vi "Check If Pixels Belong In Sector.vi"() -> (3 "FIFO Timeout?":bool)   [LabVIEW 2013]
uses:
  Globals/Pixel Location Global.vi
  Globals/Accumulated Sector Intensity.vi
  Globals/Sector Parameter Global.vi
  <vilib>/rvi/FIFO/Fifo_Resource/nirvififoEmulationReadFpgaImpl.vi
  <vilib>/rvi/DataTransferAndStorage/Container/Common/niFpgaContainerGetUniqueNameForEmu.vi
  <vilib>/rvi/FIFO/Fifo_Resource/nirvififoEmulationWriteFpgaImpl.vi
  <vilib>/rvi/DataTransferAndStorage/Container/XNode/niFpgaContainer.xnode
  <vilib>/rvi/FIFO/Fifo_Resource/nirvififoEmulationRead.vi
  <vilib>/rvi/FIFO/Fifo_Resource/nirvififoEmulationWrite.vi
panel:
  out "End of  Data?":bool
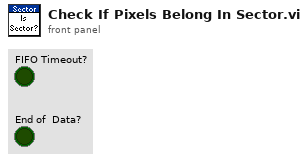
[diagram p1: front panel]
types:
  T1 = cluster{"Pixel Value":u8, "X":fxp<+,11,11>, "Y":fxp<+,11,11>}
  T2 = typedef "Sector Parameter Cluster.ctl" = cluster{"Start Angle":fxp<+/-,17,2>, "End Angle":fxp<+/-,17,2>, "Inner Radius":u16, "Outter Radius":u16, "Hinge X":u16, "Hinge Y":u16, "NumWingSectors":u8}
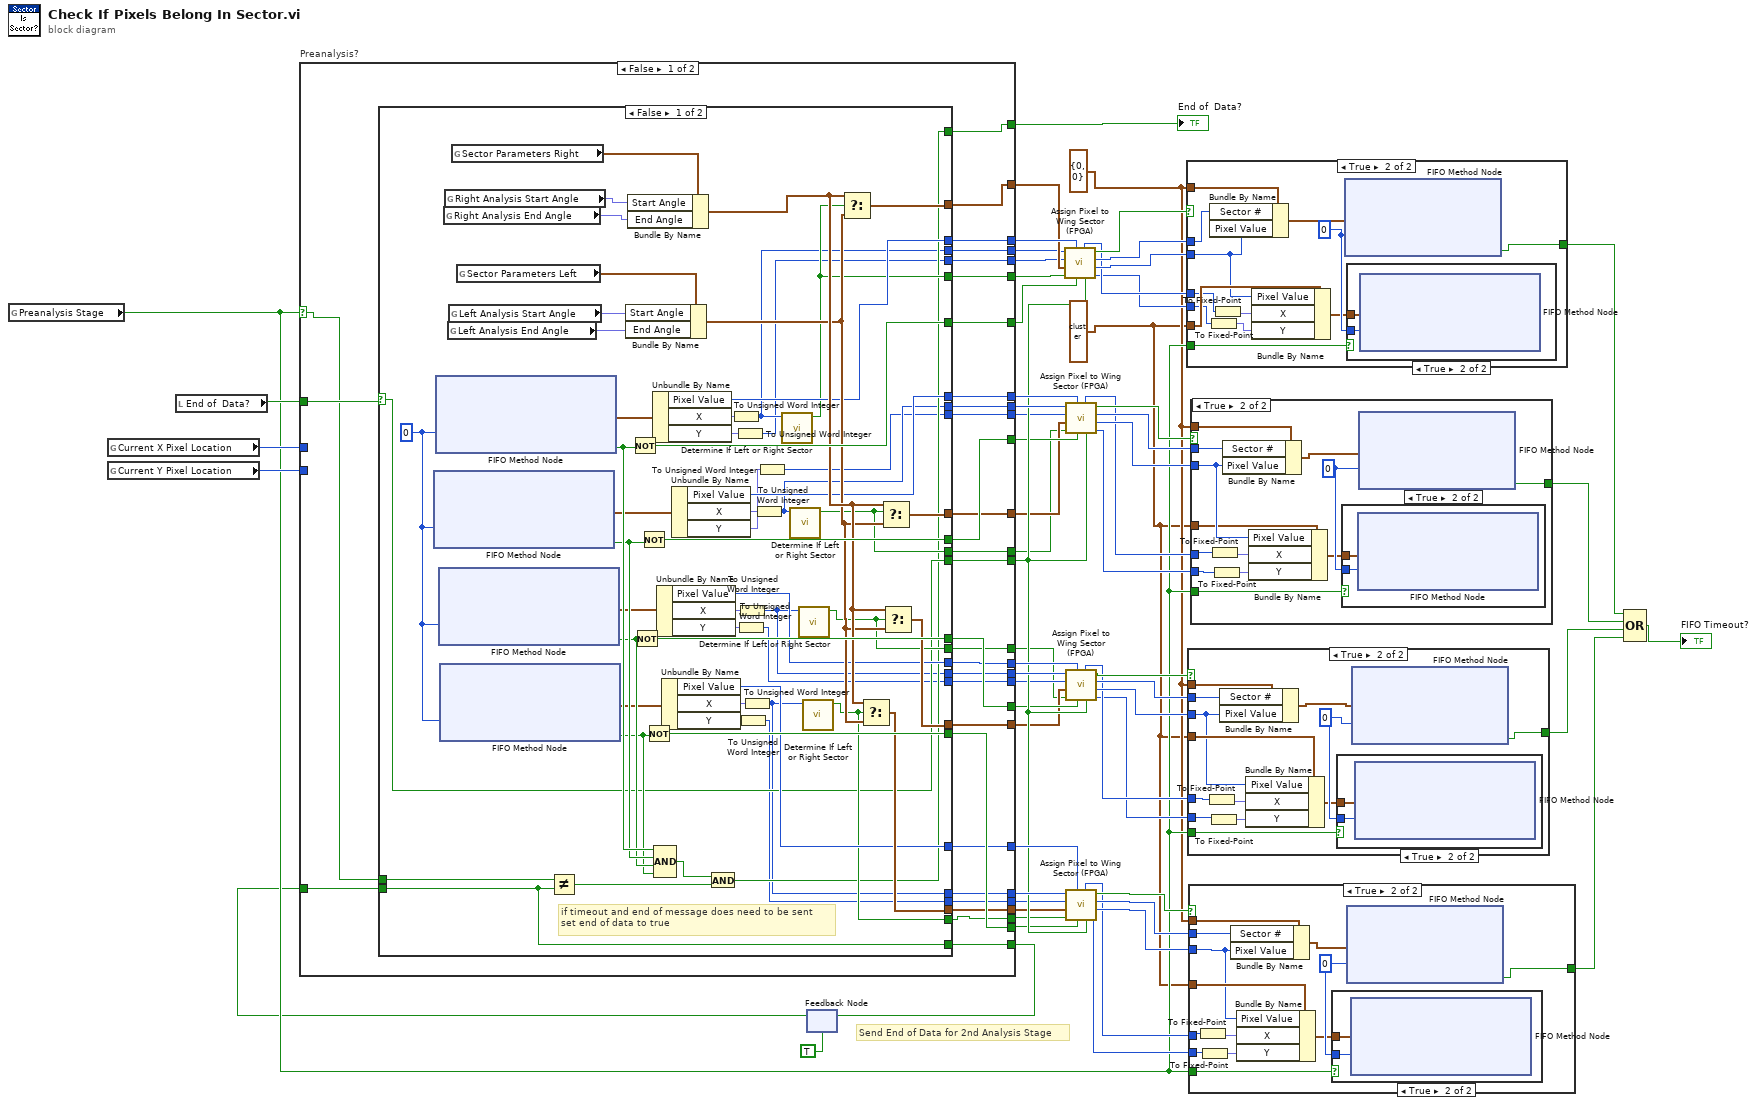
[diagram p0: block diagram]
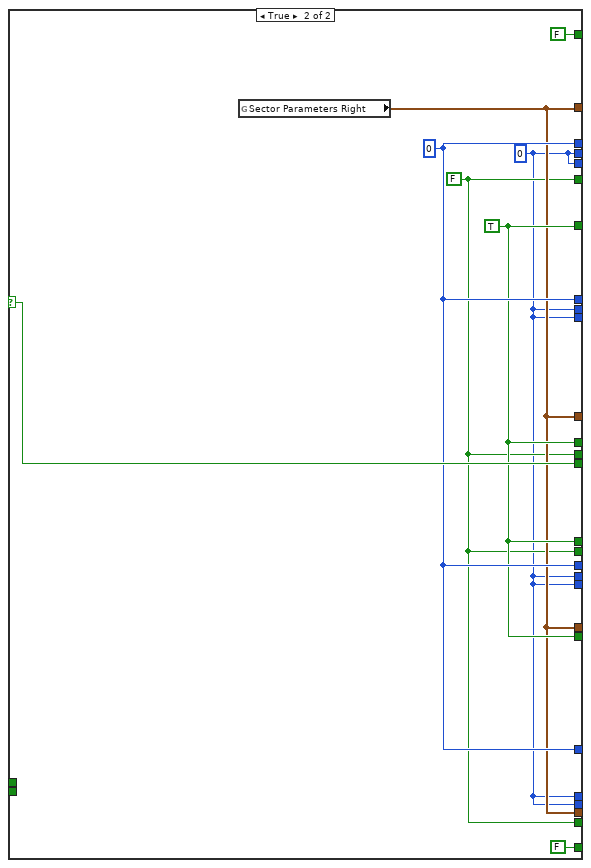
[diagram p2: hidden frame]
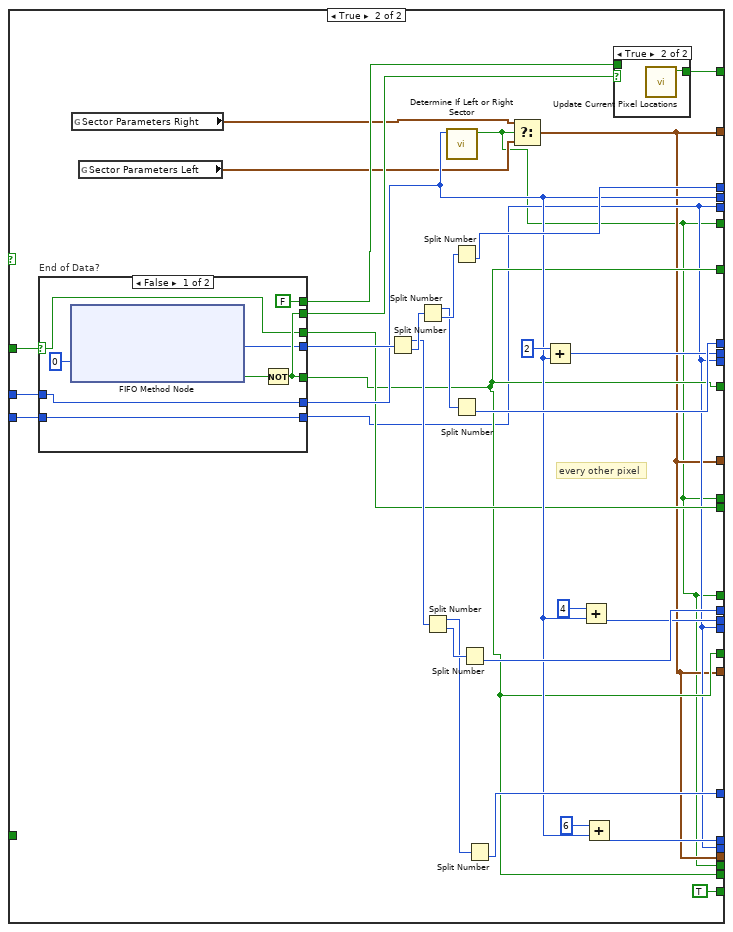
[diagram p3: hidden frame]
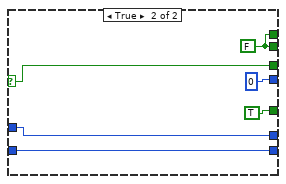
[diagram p4: hidden frame]
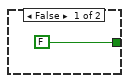
[diagram p6: hidden frame]
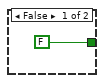
[diagram p8: hidden frame]
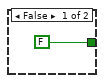
[diagram p10: hidden frame]
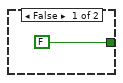
[diagram p12: hidden frame]
diagram:
  w1 = T1 {"Pixel Value"=0, "X"=0.0, "Y"=0.0} ("Element")
  w2 = cluster{"Sector #":u8, "Pixel Value":u8} {"Sector #"=0, "Pixel Value"=0} ("Element")
  # "Send End of Data for 2nd Analysis Stage"
  n1 = global read "Accumulated Sector Intensity.vi" "Preanalysis Stage"() -> (w18:bool)
  n2 = global read "Pixel Location Global.vi" "Current X Pixel Location"() -> (w29:u16)
  n3 = global read "Pixel Location Global.vi" "Current Y Pixel Location"() -> (w31:u16)
  n4 = local read "End of  Data?"() -> (w33:bool)
  n5 = feedback #1(TRUE) -> (w4:bool)
  n6 = case "Preanalysis?" shown="False" w18 {
    selector: w18 -> [w62 _]
    tunnel: [w85 w185] -> w60
    tunnel: [w67 w155] -> w42
    tunnel: [w79 w177] -> w41
    tunnel: [w78 w176] -> w40
    tunnel: [w77 w175] -> w39
    tunnel: [w76 w174] -> w38
    tunnel: [w74 w170] -> w37
    tunnel: [w73 w169] -> w36
    tunnel: [w72 w168] -> w35
    tunnel: [w83 w156] -> w34
    tunnel: [w89 w158] -> w19
    tunnel: w33 -> [w90 w165]
    tunnel: [w71 w157] -> w32
    tunnel: w31 -> [_ w164]
    tunnel: [w75 w163] -> w30
    tunnel: w29 -> [_ w162]
    tunnel: [w84 w161] -> w28
    tunnel: [w88 w158] -> w17
    tunnel: [w87 w158] -> w16
    tunnel: [w86 w158] -> w15
    tunnel: [w82 w156] -> w14
    tunnel: [w81 w156] -> w13
    tunnel: [w80 w156] -> w12
    tunnel: [w70 w157] -> w11
    tunnel: [w69 w157] -> w10
    tunnel: [w68 w157] -> w9
    tunnel: [w66 w155] -> w8
    tunnel: [w65 w155] -> w7
    tunnel: [w64 w155] -> w6
    tunnel: w4 -> [w63 _]
    tunnel: [w61 TRUE] -> w3
    frame False {
      n7 = case shown="False" w90 {
        selector: w90 -> [w108 w152]
        tunnel: [w138 w150] -> w89
        tunnel: [w137 w150] -> w88
        tunnel: [w136 w150] -> w87
        tunnel: [w135 w150] -> w86
        tunnel: [w104 FALSE] -> w85
        tunnel: [w108 w152] -> w84
        tunnel: [w130 w149] -> w83
        tunnel: [w129 w149] -> w82
        tunnel: [w128 w149] -> w81
        tunnel: [w125 w149] -> w80
        tunnel: [w124 w151] -> w79
        tunnel: [w123 w151] -> w78
        tunnel: [w122 w151] -> w77
        tunnel: [w121 w151] -> w76
        tunnel: [w102 w147] -> w75
        tunnel: [w100 w147] -> w74
        tunnel: [w98 w147] -> w73
        tunnel: [w96 w147] -> w72
        tunnel: [w101 w147] -> w71
        tunnel: [w99 w147] -> w70
        tunnel: [w97 w147] -> w69
        tunnel: [w95 w147] -> w68
        tunnel: [w112 w148] -> w67
        tunnel: [w111 w148] -> w66
        tunnel: [w110 w148] -> w65
        tunnel: [w109 w148] -> w64
        tunnel: w63 -> [w103 _]
        tunnel: w62 -> [w107 _]
        tunnel: [w103 FALSE] -> w61
        frame False {
          w139 = 0 ("Timeout")
          # "if timeout and end of message does need to be sent\nset end of data to true"
          n8 = xnode ("FIFO Method Node")("Timeout"=w139) -> ("Element"=w94:T1, "Timed Out?"=w133:bool)  [unwired: 1 in, 1 out]
          n9 = xnode ("FIFO Method Node")("Timeout"=w139) -> ("Element"=w93:T1, "Timed Out?"=w134:bool)  [unwired: 1 in, 1 out]
          n10 = xnode ("FIFO Method Node")("Timeout"=w139) -> ("Element"=w92:T1, "Timed Out?"=w132:bool)  [unwired: 1 in, 1 out]
          n11 = xnode ("FIFO Method Node")("Timeout"=w139) -> ("Element"=w91:T1, "Timed Out?"=w131:bool)  [unwired: 1 in, 1 out]
          n12 = global read "Sector Parameter Global.vi" "Right Analysis End Angle"() -> (w143:fxp<+/-,17,2>)
          n13 = global read "Sector Parameter Global.vi" "Right Analysis Start Angle"() -> (w144:fxp<+/-,17,2>)
          n14 = global read "Sector Parameter Global.vi" "Left Analysis End Angle"() -> (w140:fxp<+/-,17,2>)
          n15 = global read "Sector Parameter Global.vi" "Left Analysis Start Angle"() -> (w141:fxp<+/-,17,2>)
          n16 = global read "Sector Parameter Global.vi" "Sector Parameters Right"() -> (w145:T2)
          n17 = global read "Sector Parameter Global.vi" "Sector Parameters Left"() -> (w142:T2)
          n18 = Not Equal?(x=w107, y=w103) -> (x != y?=w105:bool)
          n19 = Bundle By Name(cluster=w142, "Start Angle"=w141, "End Angle"=w140) -> (w126:T2)
          n20 = Bundle By Name(cluster=w145, "Start Angle"=w144, "End Angle"=w143) -> (w127:T2)
          n21 = Not(x=w134) -> (.not. x?=w135:bool)
          n22 = Not(x=w132) -> (.not. x?=w137:bool)
          n23 = Not(x=w133) -> (.not. x?=w136:bool)
          n24 = Not(x=w131) -> (.not. x?=w138:bool)
          n25 = Unbundle By Name(w93) -> ("Pixel Value"=w124:u8, "X"=w120:fxp<+,11,11>, "Y"=w116:fxp<+,11,11>)
          n26 = Compound Arithmetic op=AND(w134, w133, w132, w131) -> (w106:bool)
          n27 = Unbundle By Name(w92) -> ("Pixel Value"=w122:u8, "X"=w118:fxp<+,11,11>, "Y"=w114:fxp<+,11,11>)
          n28 = Unbundle By Name(w91) -> ("Pixel Value"=w121:u8, "X"=w117:fxp<+,11,11>, "Y"=w113:fxp<+,11,11>)
          n29 = Unbundle By Name(w94) -> ("Pixel Value"=w123:u8, "X"=w119:fxp<+,11,11>, "Y"=w115:fxp<+,11,11>)
          n30 = And(x=w106, y=w105) -> (x .and. y?=w104:bool)
          n31 = To Unsigned Word Integer(number=w120) -> (unsigned 16bit integer=w102:u16)
          n32 = To Unsigned Word Integer(number=w116) -> (unsigned 16bit integer=w101:u16)
          n33 = To Unsigned Word Integer(number=w114) -> (unsigned 16bit integer=w97:u16)
          n34 = To Unsigned Word Integer(number=w118) -> (unsigned 16bit integer=w98:u16)
          n35 = To Unsigned Word Integer(number=w113) -> (unsigned 16bit integer=w95:u16)
          n36 = To Unsigned Word Integer(number=w117) -> (unsigned 16bit integer=w96:u16)
          n37 = To Unsigned Word Integer(number=w119) -> (unsigned 16bit integer=w100:u16)
          n38 = To Unsigned Word Integer(number=w115) -> (unsigned 16bit integer=w99:u16)
          n39 = call "Determine If Left or Right Sector.vi"("X Pixel Location"=w102) -> ("Right Sector?"=w112:bool)  [unwired: 10 in]
          n40 = call "Determine If Left or Right Sector.vi"("X Pixel Location"=w100) -> ("Right Sector?"=w111:bool)  [unwired: 10 in]
          n41 = call "Determine If Left or Right Sector.vi"("X Pixel Location"=w98) -> ("Right Sector?"=w110:bool)  [unwired: 10 in]
          n42 = call "Determine If Left or Right Sector.vi"("X Pixel Location"=w96) -> ("Right Sector?"=w109:bool)  [unwired: 10 in]
          n43 = Select(t=w127, s=w112, f=w126) -> (s? t:f=w130:T2)
          n44 = Select(t=w127, s=w109, f=w126) -> (s? t:f=w125:T2)
          n45 = Select(t=w127, s=w111, f=w126) -> (s? t:f=w129:T2)
          n46 = Select(t=w127, s=w110, f=w126) -> (s? t:f=w128:T2)
        }
        frame True {
          w147 = u16 0 ("X")
          w148 = FALSE ("Right Sector?")
          w150 = TRUE
          w151 = u8 0 ("Pixel Value")
          n47 = global read "Sector Parameter Global.vi" "Sector Parameters Right"() -> (w149:T2)
        }
      }
    }
    frame True {
      # "every other pixel"
      n48 = case "End of Data?" shown="False" w165 {
        selector: w165 -> [w187 w194]
        tunnel: [w191 TRUE ("Timed Out?")] -> w158
        tunnel: [w186 u64 0 ("Element")] -> w184
        tunnel: [w191 w197] -> w167
        tunnel: [FALSE ("Timed Out?") w197] -> w166
        tunnel: [w189 w195] -> w157
        tunnel: w164 -> [w189 w195]
        tunnel: [w188 w196] -> w163
        tunnel: w162 -> [w188 w196]
        tunnel: [w187 w194] -> w161
        frame False {
          n49 = xnode ("FIFO Method Node")("Timeout"=0) -> ("Element"=w186:u64, "Timed Out?"=w192:bool)  [unwired: 1 in, 1 out]
          n50 = Not(x=w192) -> (.not. x?=w191:bool)
        }
        frame True {
          w197 = FALSE ("Timed Out?")
        }
      }
      n51 = global read "Sector Parameter Global.vi" "Sector Parameters Right"() -> (w160:T2)
      n52 = global read "Sector Parameter Global.vi" "Sector Parameters Left"() -> (w159:T2)
      n53 = Split Number(x=w184) -> (hi(x)=w182:u32, lo(x)=w183:u32)
      n54 = Split Number(x=w183) -> (hi(x)=w180:u16, lo(x)=w181:u16)
      n55 = Split Number(x=w182) -> (hi(x)=w178:u16, lo(x)=w179:u16)
      n56 = call "Determine If Left or Right Sector.vi"("X Pixel Location"=w163) -> ("Right Sector?"=w155:bool)  [unwired: 10 in]
      n57 = Split Number(x=w181) -> (lo(x)=w177:u8)  [unwired: 1 out]
      n58 = Split Number(x=w180) -> (lo(x)=w176:u8)  [unwired: 1 out]
      n59 = Split Number(x=w179) -> (lo(x)=w175:u8)  [unwired: 1 out]
      n60 = Split Number(x=w178) -> (lo(x)=w174:u8)  [unwired: 1 out]
      n61 = Select(t=w160, s=w155, f=w159) -> (s? t:f=w156:T2)
      n62 = Add(x=u16 2, y=w163) -> (x+y=w170:u16)
      n63 = Add(x=u16 4, y=w163) -> (x+y=w169:u16)
      n64 = Add(x=u16 6, y=w163) -> (x+y=w168:u16)
      n65 = case shown="True" w167 {
        tunnel: [w200 w201] -> w185
        tunnel: w166 -> [w200 _]
        frame False {
        }
        frame True {
          n66 = call "Update Current Pixel Locations.vi"() -> ("End of data?"=w201:bool)  [unwired: 11 in]
        }
      }
    }
  }
  "End of  Data?" <- w60
  n67 = feedback-in #1(w3) -> ()
  n68 = call "Assign Pixel to Wing Sector (FPGA).vi"("End of Data?"=w28, "Valid Data?"=w15, "Pixel Intensity In"=w41, "Right Wing?"=w42, "Sector Parameters"=w34, "Pixel Y"=w32, "Pixel X"=w30) -> ("Y"=w26:u16, "Pixel Intensity Out"=w52:u8, "sector #"=w53:u8, "output valid"=w54:bool, "X"=w27:u16)
  n69 = call "Assign Pixel to Wing Sector (FPGA).vi"("End of Data?"=w28, "Valid Data?"=w16, "Pixel Intensity In"=w40, "Right Wing?"=w8, "Sector Parameters"=w14, "Pixel Y"=w11, "Pixel X"=w37) -> ("Y"=w24:u16, "Pixel Intensity Out"=w49:u8, "sector #"=w50:u8, "output valid"=w51:bool, "X"=w25:u16)
  n70 = call "Assign Pixel to Wing Sector (FPGA).vi"("End of Data?"=w28, "Valid Data?"=w17, "Pixel Intensity In"=w39, "Right Wing?"=w7, "Sector Parameters"=w13, "Pixel Y"=w10, "Pixel X"=w36) -> ("Y"=w22:u16, "Pixel Intensity Out"=w46:u8, "sector #"=w47:u8, "output valid"=w48:bool, "X"=w23:u16)
  n71 = call "Assign Pixel to Wing Sector (FPGA).vi"("End of Data?"=w28, "Valid Data?"=w19, "Pixel Intensity In"=w38, "Right Wing?"=w6, "Sector Parameters"=w12, "Pixel Y"=w9, "Pixel X"=w35) -> ("Y"=w20:u16, "Pixel Intensity Out"=w43:u8, "sector #"=w44:u8, "output valid"=w45:bool, "X"=w21:u16)
  n72 = case shown="True" w54 {
    tunnel: w2 -> [_ w212]
    tunnel: [FALSE ("Timed Out?") w214] -> w58
    tunnel: w53 -> [_ w211]
    tunnel: w52 -> [_ w209]
    tunnel: w27 -> [_ w207]
    tunnel: w26 -> [_ w205]
    tunnel: w18 -> [_ w213]
    tunnel: w1 -> [_ w210]
    frame False {
    }
    frame True {
      w215 = 0 ("Timeout")
      n73 = To Fixed-Point(number=w205) -> (fixed-point=w204:fxp<+,11,11>)  [unwired: 1 in]
      n74 = Bundle By Name(cluster=w212, "Sector #"=w211, "Pixel Value"=w209) -> (w203:cluster{"Sector #":u8, "Pixel Value":u8})
      n75 = To Fixed-Point(number=w207) -> (fixed-point=w206:fxp<+,11,11>)  [unwired: 1 in]
      n76 = Bundle By Name(cluster=w210, "Pixel Value"=w209, "X"=w206, "Y"=w204) -> (w208:T1)
      n77 = xnode ("FIFO Method Node")("Element"=w203, "Timeout"=w215) -> ("Timed Out?"=w214:bool)  [unwired: 1 in, 1 out]
      n78 = case shown="True" w213 {
        tunnel: w215 -> [_ w217]
        tunnel: w208 -> [_ w216]
        frame False {
        }
        frame True {
          n79 = xnode ("FIFO Method Node")("Element"=w216, "Timeout"=w217) -> ()  [unwired: 1 in, 2 out]
        }
      }
    }
  }
  n80 = case shown="True" w48 {
    tunnel: w2 -> [_ w229]
    tunnel: [FALSE ("Timed Out?") w231] -> w56
    tunnel: w47 -> [_ w228]
    tunnel: w46 -> [_ w220]
    tunnel: w23 -> [_ w222]
    tunnel: w22 -> [_ w221]
    tunnel: w18 -> [_ w227]
    tunnel: w1 -> [_ w224]
    frame False {
    }
    frame True {
      w230 = 0 ("Timeout")
      n81 = To Fixed-Point(number=w222) -> (fixed-point=w226:fxp<+,11,11>)  [unwired: 1 in]
      n82 = To Fixed-Point(number=w221) -> (fixed-point=w225:fxp<+,11,11>)  [unwired: 1 in]
      n83 = Bundle By Name(cluster=w229, "Sector #"=w228, "Pixel Value"=w220) -> (w219:cluster{"Sector #":u8, "Pixel Value":u8})
      n84 = Bundle By Name(cluster=w224, "Pixel Value"=w220, "X"=w226, "Y"=w225) -> (w223:T1)
      n85 = case shown="True" w227 {
        tunnel: w230 -> [_ w233]
        tunnel: w223 -> [_ w232]
        frame False {
        }
        frame True {
          n86 = xnode ("FIFO Method Node")("Element"=w232, "Timeout"=w233) -> ()  [unwired: 1 in, 2 out]
        }
      }
      n87 = xnode ("FIFO Method Node")("Element"=w219, "Timeout"=w230) -> ("Timed Out?"=w231:bool)  [unwired: 1 in, 1 out]
    }
  }
  n88 = case shown="True" w45 {
    tunnel: w2 -> [_ w245]
    tunnel: [FALSE ("Timed Out?") w246] -> w55
    tunnel: w44 -> [_ w244]
    tunnel: w43 -> [_ w239]
    tunnel: w21 -> [_ w238]
    tunnel: w20 -> [_ w237]
    tunnel: w18 -> [_ w243]
    tunnel: w1 -> [_ w240]
    frame False {
    }
    frame True {
      w247 = 0 ("Timeout")
      n89 = To Fixed-Point(number=w238) -> (fixed-point=w241:fxp<+,11,11>)  [unwired: 1 in]
      n90 = To Fixed-Point(number=w237) -> (fixed-point=w242:fxp<+,11,11>)  [unwired: 1 in]
      n91 = Bundle By Name(cluster=w245, "Sector #"=w244, "Pixel Value"=w239) -> (w235:cluster{"Sector #":u8, "Pixel Value":u8})
      n92 = Bundle By Name(cluster=w240, "Pixel Value"=w239, "X"=w241, "Y"=w242) -> (w236:T1)
      n93 = case shown="True" w243 {
        tunnel: w247 -> [_ w249]
        tunnel: w236 -> [_ w248]
        frame False {
        }
        frame True {
          n94 = xnode ("FIFO Method Node")("Element"=w248, "Timeout"=w249) -> ()  [unwired: 1 in, 2 out]
        }
      }
      n95 = xnode ("FIFO Method Node")("Element"=w235, "Timeout"=w247) -> ("Timed Out?"=w246:bool)  [unwired: 1 in, 1 out]
    }
  }
  n96 = case shown="True" w51 {
    tunnel: w2 -> [_ w261]
    tunnel: [FALSE ("Timed Out?") w262] -> w57
    tunnel: w50 -> [_ w260]
    tunnel: w49 -> [_ w256]
    tunnel: w25 -> [_ w254]
    tunnel: w24 -> [_ w255]
    tunnel: w18 -> [_ w259]
    tunnel: w1 -> [_ w253]
    frame False {
    }
    frame True {
      w263 = 0 ("Timeout")
      n97 = To Fixed-Point(number=w254) -> (fixed-point=w257:fxp<+,11,11>)  [unwired: 1 in]
      n98 = To Fixed-Point(number=w255) -> (fixed-point=w258:fxp<+,11,11>)  [unwired: 1 in]
      n99 = Bundle By Name(cluster=w261, "Sector #"=w260, "Pixel Value"=w256) -> (w251:cluster{"Sector #":u8, "Pixel Value":u8})
      n100 = Bundle By Name(cluster=w253, "Pixel Value"=w256, "X"=w257, "Y"=w258) -> (w252:T1)
      n101 = case shown="True" w259 {
        tunnel: w263 -> [_ w265]
        tunnel: w252 -> [_ w264]
        frame False {
        }
        frame True {
          n102 = xnode ("FIFO Method Node")("Element"=w264, "Timeout"=w265) -> ()  [unwired: 1 in, 2 out]
        }
      }
      n103 = xnode ("FIFO Method Node")("Element"=w251, "Timeout"=w263) -> ("Timed Out?"=w262:bool)  [unwired: 1 in, 1 out]
    }
  }
  n104 = Compound Arithmetic op=OR(w58, w57, w56, w55) -> (→"FIFO Timeout?":bool)
